vi "Process.vi"(9 "Module Info In":T1, 11 "Engine Tags In":T3) -> (1 "Module Info Out":T1, 3 "Engine Tags Out":T3)   [LabVIEW 2013, in "synchronous engine runtime.lvclass"]
uses:
  synchronous engine runtime.lvclass
  <vilib>/NI/Tag Bus/table/data table.ctl
  Module Execution Info.ctl
  <vilib>/NI/Tag Bus Module Framework/runtime/TBM module execution interface.lvclass
  Data Table with Transfer Spec.ctl
  <vilib>/NI/Tag Bus/table/transfer specification.ctl
  <vilib>/NI/Tag Bus/tag/Data Type.ctl
  <vilib>/NI/Tag Bus/table/data table.lvlib
  <vilib>/NI/Tag Bus/tag/tag descriptor.lvclass
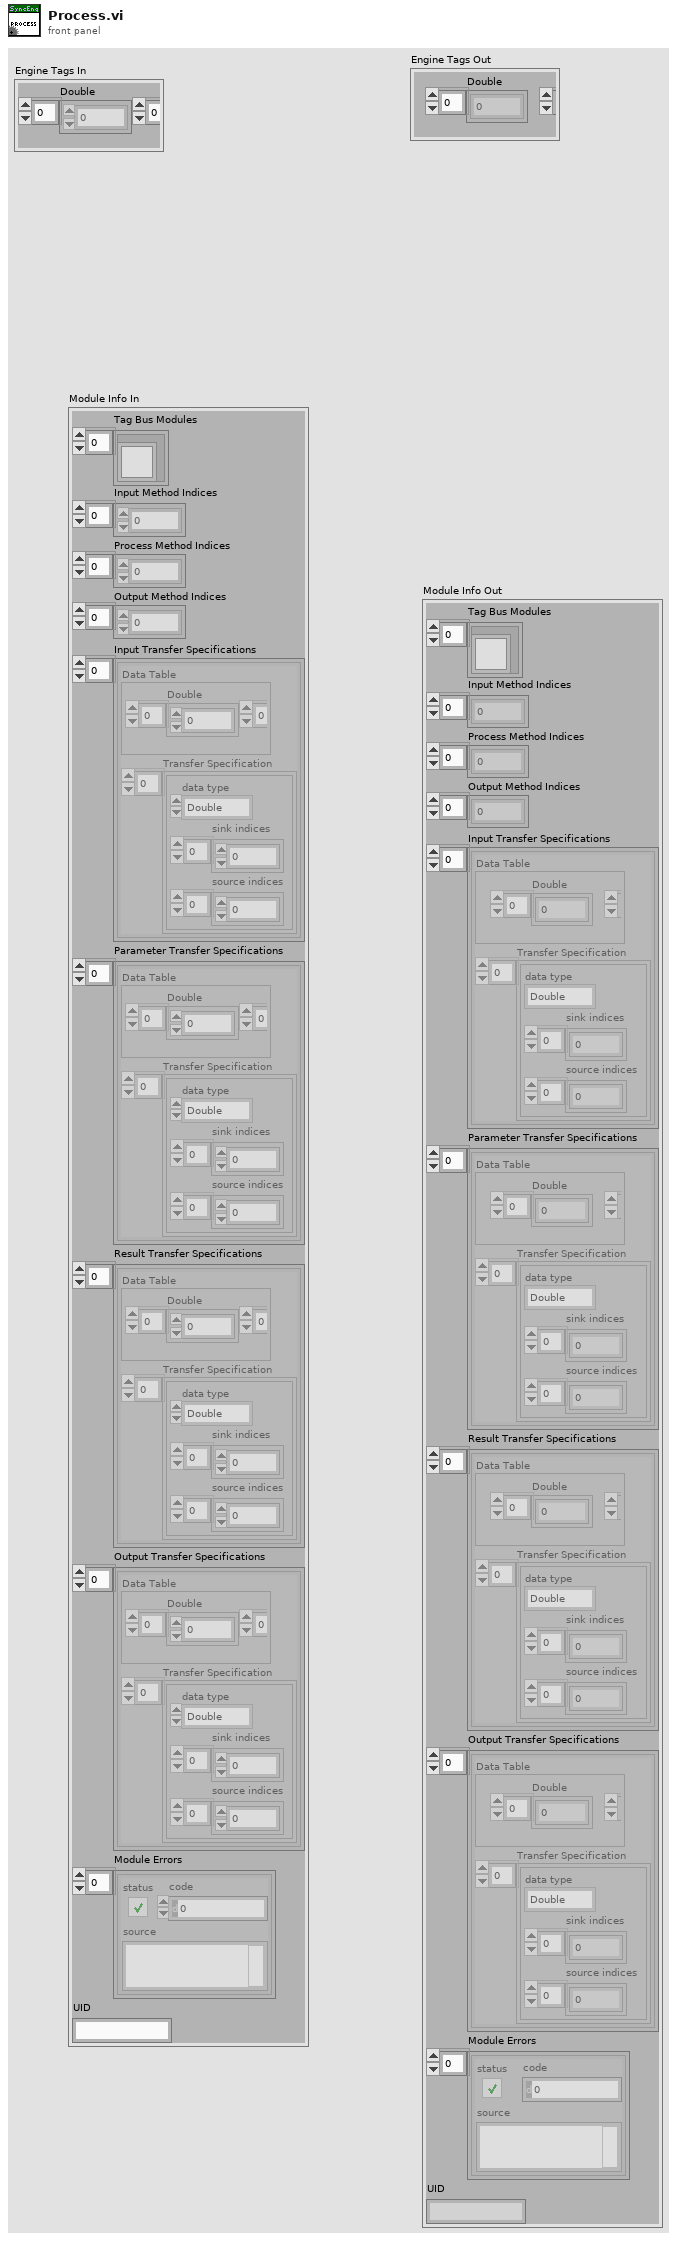
[diagram p1: front panel]
types:
  T1 = typedef "synchronous engine runtime.lvclass/Module Execution Info.ctl" = cluster{"Tag Bus Modules":refnum<class "TBM module execution interface.lvclass">[], "Input Method Indices":i32[], "Process Method Indices":i32[], "Output Method Indices":i32[], "Input Transfer Specifications":T2[], "Parameter Transfer Specifications":T2[], "Result Transfer Specifications":T2[], "Output Transfer Specifications":T2[], "Module Errors":errorcluster[], "UID":string}
  T2 = typedef "synchronous engine runtime.lvclass/Data Table with Transfer Spec.ctl" = cluster{"Data Table":T3, "Transfer Specification":T4[]}
  T3 = typedef "tag bus.lvlib/data table.lvlib/data table.ctl" = cluster{"Double":dbl[], "Single":sgl[], "I64":i64[], "I32":i32[], "I16":i16[], "I8":i8[], "U64":u64[], "U32":u32[], "U16":u16[], "U8":u8[], "Boolean":bool[], "String":string[], "Array of Double":cluster{"DBL Array":dbl[]}[], "Array of Single":cluster{"SGL Array":sgl[]}[], "Array of I64":cluster{"I64 Array":i64[]}[], "Array of I32":cluster{"I32 Array":i32[]}[], "Array of I16":cluster{"I16 Array":i16[]}[], "Array of I8":cluster{"I8 Array":i8[]}[], "Array of U64":cluster{"U64 Array":u64[]}[], "Array of U32":cluster{"U32 Array":u32[]}[], "Array of U16":cluster{"U16 Array":u16[]}[], "Array of U8":cluster{"U8 Array":u8[]}[], "Array of Boolean":cluster{"Boolean Array":bool[]}[], "Array of String":cluster{"String Array":string[]}[]}
  T4 = typedef "tag bus.lvlib/data table.lvlib/transfer specification.ctl" = cluster{"data type":T5, "sink indices":i32[], "source indices":i32[]}
  T5 = typedef "tag bus.lvlib/tag descriptor.lvclass/Data Type.ctl" = enum16{"Double", "Single", "I64", "I32", "I16", "I8", "U64", "U32", "U16", "U8", "Boolean", "String", "Array of Double", "Array of Single", "Array of I64", "Array of I32", "Array of I16", "Array of I8", "Array of U64", "Array of U32", "Array of U16", "Array of U8", "Array of Boolean", "Array of String"}
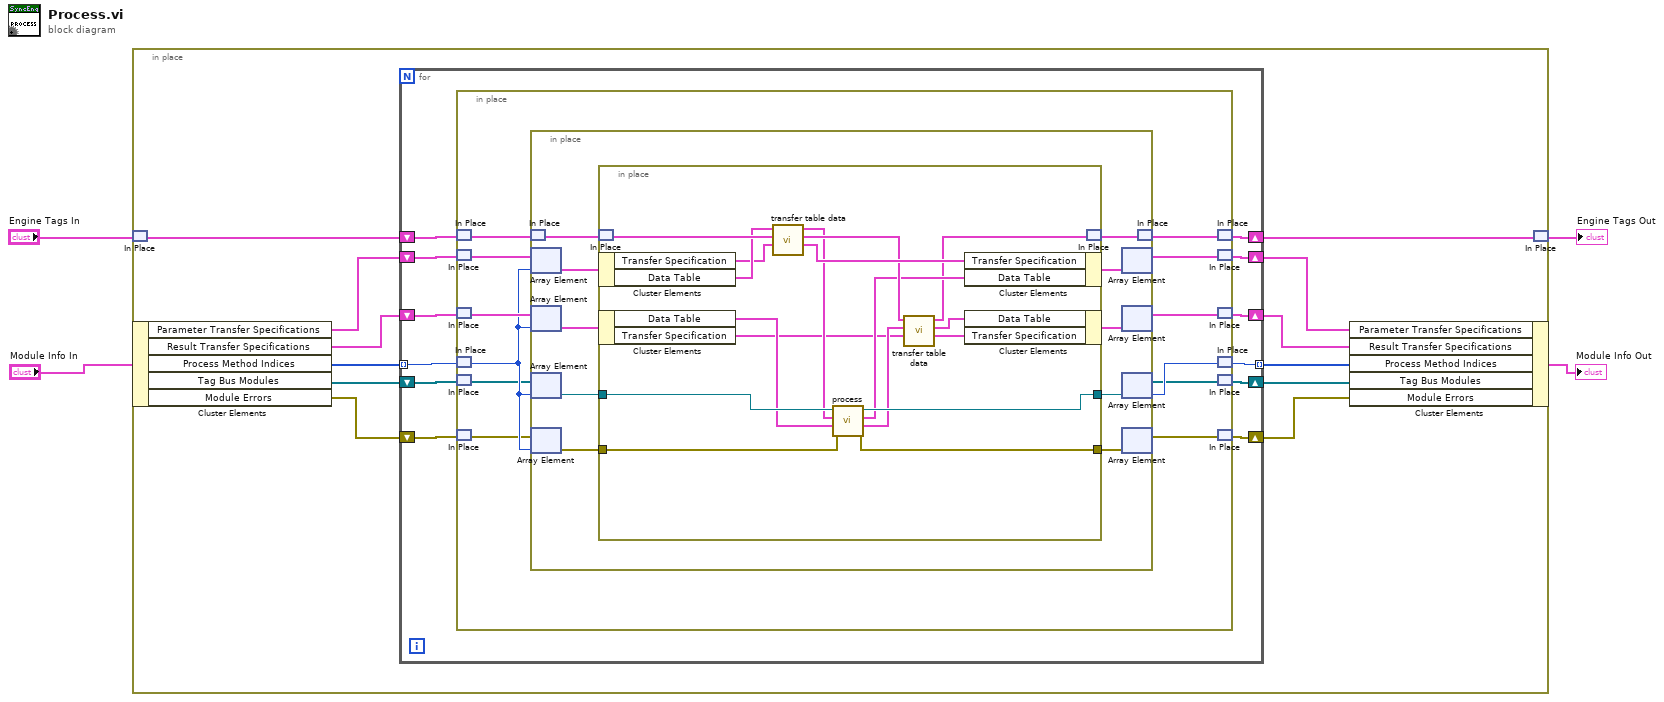
[diagram p0: block diagram]
diagram:
  n1 = in-place {
    n2 = in-place-match #1("Engine Tags In") -> (w16:T3)
    n3 = in-place-cluster #2("Module Info In") -> ("Parameter Transfer Specifications"=w14:T2[], "Result Transfer Specifications"=w11:T2[], "Process Method Indices"=w7:i32[], "Tag Bus Modules"=w8:refnum<class "TBM module execution interface.lvclass">[], "Module Errors"=w13:errorcluster[])
    n4 = for {
      shift-right: [w19] -> w5
      shift-left: w8 -> [w20]
      shift-right: [w27] -> w15
      shift-left: w16 -> [w28]
      shift-right: [w25] -> w10
      shift-left: w14 -> [w26]
      shift-right: [w17] -> w12
      shift-left: w13 -> [w18]
      shift-right: [w23] -> w9
      shift-left: w11 -> [w24]
      tunnel: [w21] -> w6 mode=indexing
      tunnel: w7 -> [w22] mode=indexing
      n5 = in-place {
        n6 = in-place-match #3(w28) -> (w40:T3)
        n7 = in-place-match #4(w26) -> (w38:T2[])
        n8 = in-place-match #5(w24) -> (w36:T2[])
        n9 = in-place-match #6(w22) -> (w34:i32)
        n10 = in-place-match #7(w20) -> (w32:refnum<class "TBM module execution interface.lvclass">[])
        n11 = in-place-match #8(w18) -> (w30:errorcluster[])
        n12 = in-place {
          n13 = in-place-match #9(w40) -> (w46:T3)
          n14 = in-place-array #10(w38, w34) -> (w44:T2)
          n15 = in-place-array #11(w36, w34) -> (w43:T2)
          n16 = in-place-array #12(w32, w34) -> (w50:refnum<class "TBM module execution interface.lvclass">)
          n17 = in-place-array #13(w30, w34) -> (w48:errorcluster)
          n18 = in-place {
            in-place-border: w50 -> [w67]
            in-place-border: [w66] -> w49
            in-place-border: w48 -> [w65]
            in-place-border: [w64] -> w47
            n19 = in-place-match #14(w46) -> (w63:T3)
            n20 = in-place-cluster #15(w44) -> ("Transfer Specification"=w61:T4[], "Data Table"=w62:T3)
            n21 = in-place-cluster #16(w43) -> ("Data Table"=w57:T3, "Transfer Specification"=w54:T4[])
            n22 = call <vilib>:"transfer table data.vi"("transfer specification in"=w61, "data table source in"=w63, "data table sink in"=w62) -> ("transfer specification out"=w60:T4[], "data table source out"=w59:T3, "data table sink out"=w58:T3)  [unwired: 6 in]
            n23 = call-dynamic "process.vi"("error in"=w65, "result allocation"=w57, "parameters"=w58, "module in"=w67) -> ("error out"=w64:errorcluster, "results"=w55:T3, "parameter allocation"=w56:T3, "module out"=w66:refnum<class "TBM module execution interface.lvclass">)  [unwired: 4 in]
            n24 = call <vilib>:"transfer table data.vi"("transfer specification in"=w54, "data table source in"=w55, "data table sink in"=w59) -> ("transfer specification out"=w53:T4[], "data table source out"=w52:T3, "data table sink out"=w51:T3)  [unwired: 6 in]
            n25 = in-place-cluster #15("Transfer Specification"=w60, "Data Table"=w56) -> (w41:T2)
            n26 = in-place-cluster #16("Data Table"=w52, "Transfer Specification"=w53) -> (w42:T2)
            n27 = in-place-match #14(w51) -> (w45:T3)
          }
          n28 = in-place-array #10(w41) -> (w37:T2[])  [unwired: 1 out]
          n29 = in-place-array #11(w42) -> (w35:T2[])  [unwired: 1 out]
          n30 = in-place-array #12(w49) -> (w31:refnum<class "TBM module execution interface.lvclass">[], w33:i32)
          n31 = in-place-array #13(w47) -> (w29:errorcluster[])  [unwired: 1 out]
          n32 = in-place-match #9(w45) -> (w39:T3)
        }
        n33 = in-place-match #3(w39) -> (w27:T3)
        n34 = in-place-match #4(w37) -> (w25:T2[])
        n35 = in-place-match #5(w35) -> (w23:T2[])
        n36 = in-place-match #6(w33) -> (w21:i32)
        n37 = in-place-match #7(w31) -> (w19:refnum<class "TBM module execution interface.lvclass">[])
        n38 = in-place-match #8(w29) -> (w17:errorcluster[])
      }
    }
    n39 = in-place-cluster #2("Parameter Transfer Specifications"=w10, "Result Transfer Specifications"=w9, "Process Method Indices"=w6, "Tag Bus Modules"=w5, "Module Errors"=w12) -> (→"Module Info Out":T1)
    n40 = in-place-match #1(w15) -> (→"Engine Tags Out":T3)
  }
